vi "Set Digital Output.vi"(8 "error in (no error)":errorcluster, 9 "Value":bool, 10 "Channel":i32, 11 "VISA resource name in":refnum<visa-resource-name>) -> (0 "error out":errorcluster, 3 "VISA resource name":refnum<visa-resource-name>)   [LabVIEW 2020, in "CTI-Visa.lvlib"]
uses:
  CTI-Visa.lvlib
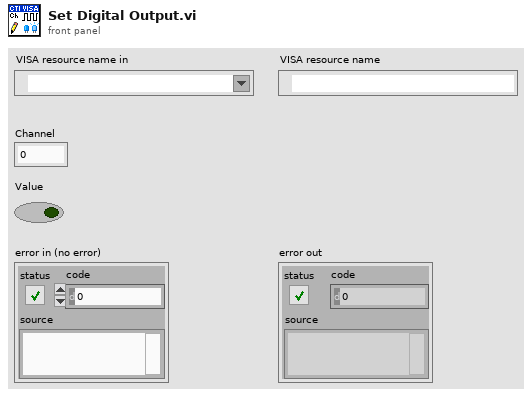
[diagram p1: front panel]
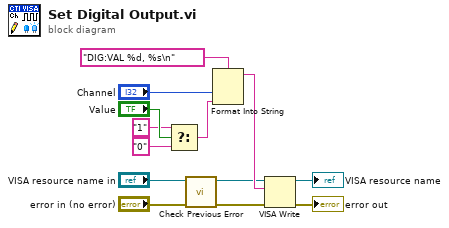
[diagram p0: block diagram]
diagram:
  n1 = Select(t="1", s="Value", f="0") -> (s? t:f=w8:string)
  n2 = call "Check Previous Error.vi"("error in (no error)"="error in (no error)", "VISA resource name in"="VISA resource name in") -> ("error out"=w1:errorcluster, "VISA resource name"=w3:refnum<visa-resource-name>)  [unwired: 8 in]
  n3 = Format Into String(format string="DIG:VAL %d, %s\n", "Channel", w8) -> (resulting string=w6:string)  [unwired: 2 in, 1 out]
  n4 = VISA Write(VISA resource name=w3, write buffer=w6, error in (no error)=w1) -> (VISA resource name out=→"VISA resource name":refnum<visa-resource-name>, error out=→"error out":errorcluster)  [unwired: 1 out]
